vi "test lvjson set.vi"(8 "error in (no error)":errorcluster) -> (0 "error out":errorcluster)   [LabVIEW 2019, in "labview_json_tests.lvlib"]
uses:
  labview_json_tests.lvlib
  lib/Element Set Behavior.ctl
  lib/labview_json.lvlib
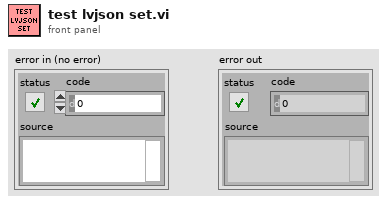
[diagram p1: front panel]
types:
  T1 = typedef "labview_json.lvlib/Element Set Behavior.ctl" = enum8{"Add or Modify", "Modify Only", "Replace"}
  T2 = cluster{"homeTown":string, "formed":i32, "members":cluster{"age":u64}[]}
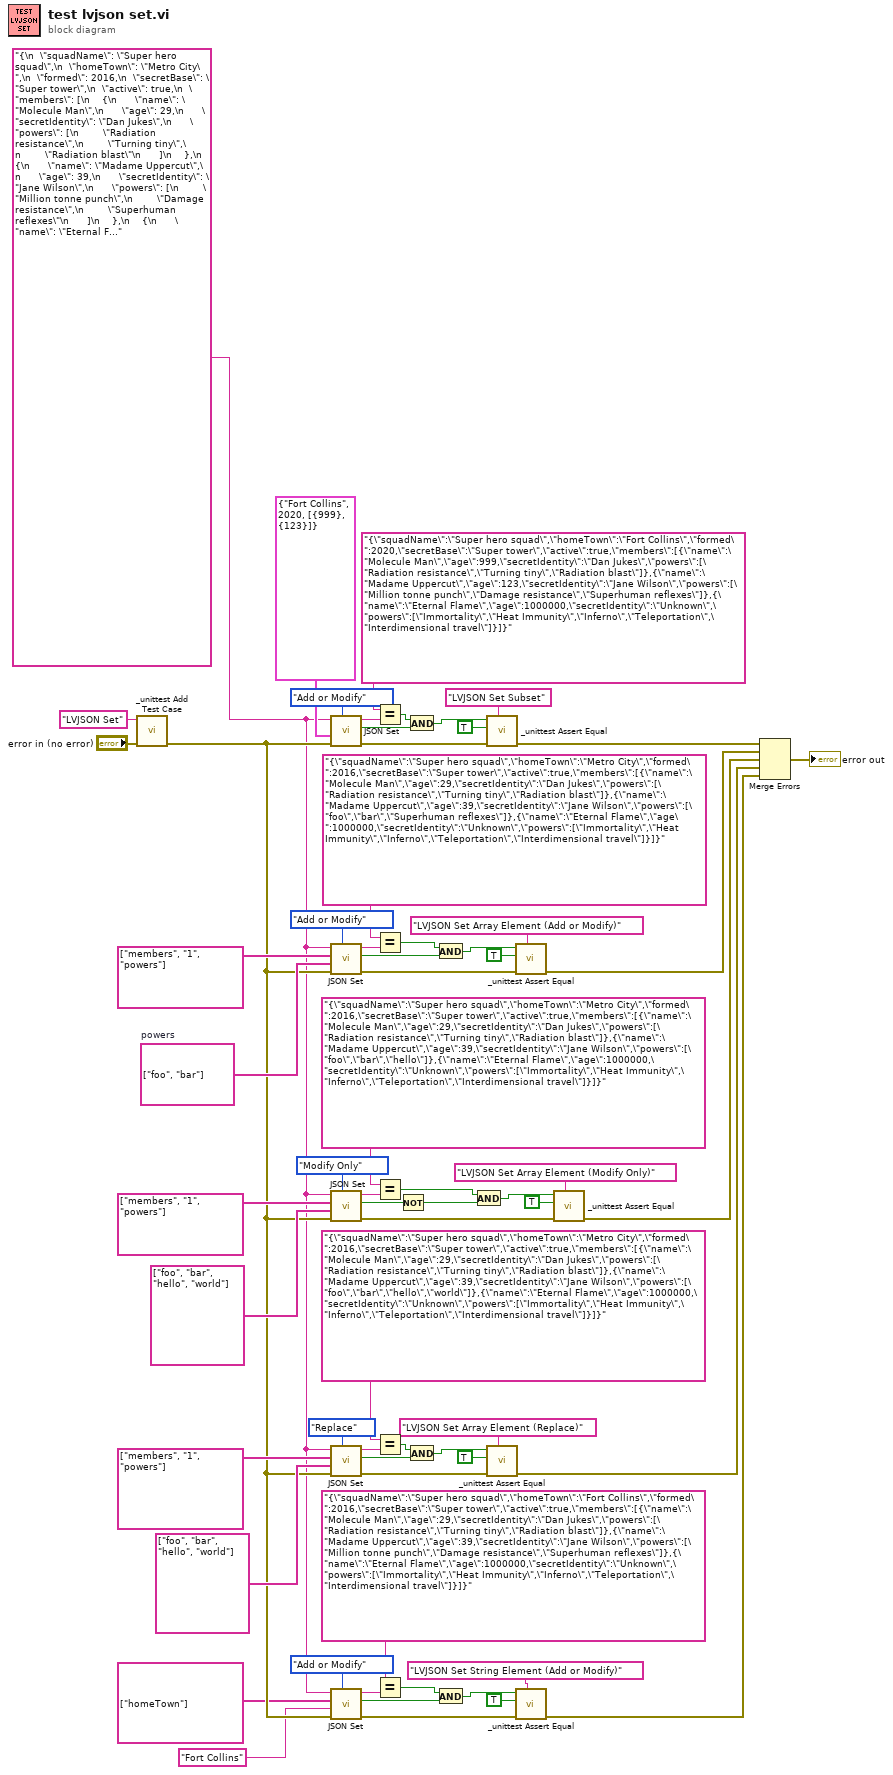
[diagram p0: block diagram]
diagram:
  w15 = string[] ["foo", "bar"]  # powers
  w3 = "{\n  \"squadName\": \"Super hero squad\",\n  \"homeTown\": \"Metro City\",\n  \"formed\": 2016,\n  \"secretBase\": \"Super tower\",\n  \"active\": true,\n  \"members\": [\n    {\n      \"name\": \"Molecule Man\",\n      \"age\": 29,\n      \"secretIdentity\": \"Dan Jukes\",\n      \"powers\": [\n        \"Radiation resistance\",\n        \"Turning tiny\",\n        \"Radiation blast\"\n      ]\n    },\n    {\n      \"name\": \"Madame Uppercut\",\n      \"age\": 39,\n      \"secretIdentity\": \"Jane Wilson\",\n      \"powers\": [\n        \"Million tonne punch\",\n        \"Damage resistance\",\n        \"Superhuman reflexes\"\n      ]\n    },\n    {\n      \"name\": \"Eternal Flame\",\n      \"age\": 1000000,\n      \"secretIdentity\": \"Unknown\",\n      \"powers\": [\n        \"Immortality\",\n        \"Heat Immunity\",\n        \"Inferno\",\n        \"Teleportation\",\n        \"Interdimensional travel\"\n      ]\n    }\n  ]\n}"
  n1 = call "_unittest Add Test Case.vi"("error in (no error)"="error in (no error)", "Test Case"="LVJSON Set") -> ("error out"=w6:errorcluster)  [unwired: 9 in]
  n2 = call "JSON Set.vi"("Behavior (Add or Modify)"=Element_Set_Behavior."Add or Modify", "error in (no error)"=w6, "Value"=T2 {"homeTown"="Fort Collins", "formed"=2020, "members"=[{"age"=999}, {"age"=123}]} ("Root"), "JSON in"=w3) -> ("error out"=w54:errorcluster, "Exists?"=w53:bool, "JSON out"=w56:string)  [unwired: 5 in]
  n3 = call "JSON Set.vi"("Behavior (Add or Modify)"=Element_Set_Behavior."Add or Modify", "error in (no error)"=w6, "Value"=w15, "Root Path ([]=Root)"=string[] ["members", "1", "powers"] ("x"), "JSON in"=w3) -> ("error out"=w51:errorcluster, "Exists?"=w52:bool, "JSON out"=w50:string)  [unwired: 4 in]
  n4 = call "JSON Set.vi"("Behavior (Add or Modify)"=Element_Set_Behavior."Modify Only", "error in (no error)"=w6, "Value"=string[] ["foo", "bar", "hello", "world"], "Root Path ([]=Root)"=string[] ["members", "1", "powers"] ("x"), "JSON in"=w3) -> ("error out"=w32:errorcluster, "Exists?"=w31:bool, "JSON out"=w33:string)  [unwired: 4 in]
  n5 = call "JSON Set.vi"("Behavior (Add or Modify)"=Element_Set_Behavior."Replace", "error in (no error)"=w6, "Value"=string[] ["foo", "bar", "hello", "world"], "Root Path ([]=Root)"=string[] ["members", "1", "powers"] ("x"), "JSON in"=w3) -> ("error out"=w28:errorcluster, "Exists?"=w29:bool, "JSON out"=w27:string)  [unwired: 4 in]
  n6 = call "JSON Set.vi"("Behavior (Add or Modify)"=Element_Set_Behavior."Add or Modify", "error in (no error)"=w6, "Value"="Fort Collins", "Root Path ([]=Root)"=string[] ["homeTown"] ("x"), "JSON in"=w3) -> ("error out"=w8:errorcluster, "Exists?"=w7:bool, "JSON out"=w9:string)  [unwired: 4 in]
  n7 = Equal?(x="{\"squadName\":\"Super hero squad\",\"homeTown\":\"Fort Collins\",\"formed\":2020,\"secretBase\":\"Super tower\",\"active\":true,\"members\":[{\"name\":\"Molecule Man\",\"age\":999,\"secretIdentity\":\"Dan Jukes\",\"powers\":[\"Radiation resistance\",\"Turning tiny\",\"Radiation blast\"]},{\"name\":\"Madame Uppercut\",\"age\":123,\"secretIdentity\":\"Jane Wilson\",\"powers\":[\"Million tonne punch\",\"Damage resistance\",\"Superhuman reflexes\"]},{\"name\":\"Eternal Flame\",\"age\":1000000,\"secretIdentity\":\"Unknown\",\"powers\":[\"Immortality\",\"Heat Immunity\",\"Inferno\",\"Teleportation\",\"Interdimensional travel\"]}]}" ("JSON"), y=w56) -> (x = y?=w59:bool)
  n8 = Equal?(x="{\"squadName\":\"Super hero squad\",\"homeTown\":\"Metro City\",\"formed\":2016,\"secretBase\":\"Super tower\",\"active\":true,\"members\":[{\"name\":\"Molecule Man\",\"age\":29,\"secretIdentity\":\"Dan Jukes\",\"powers\":[\"Radiation resistance\",\"Turning tiny\",\"Radiation blast\"]},{\"name\":\"Madame Uppercut\",\"age\":39,\"secretIdentity\":\"Jane Wilson\",\"powers\":[\"foo\",\"bar\",\"Superhuman reflexes\"]},{\"name\":\"Eternal Flame\",\"age\":1000000,\"secretIdentity\":\"Unknown\",\"powers\":[\"Immortality\",\"Heat Immunity\",\"Inferno\",\"Teleportation\",\"Interdimensional travel\"]}]}" ("JSON"), y=w50) -> (x = y?=w48:bool)
  n9 = Equal?(x="{\"squadName\":\"Super hero squad\",\"homeTown\":\"Metro City\",\"formed\":2016,\"secretBase\":\"Super tower\",\"active\":true,\"members\":[{\"name\":\"Molecule Man\",\"age\":29,\"secretIdentity\":\"Dan Jukes\",\"powers\":[\"Radiation resistance\",\"Turning tiny\",\"Radiation blast\"]},{\"name\":\"Madame Uppercut\",\"age\":39,\"secretIdentity\":\"Jane Wilson\",\"powers\":[\"foo\",\"bar\",\"hello\"]},{\"name\":\"Eternal Flame\",\"age\":1000000,\"secretIdentity\":\"Unknown\",\"powers\":[\"Immortality\",\"Heat Immunity\",\"Inferno\",\"Teleportation\",\"Interdimensional travel\"]}]}" ("JSON"), y=w33) -> (x = y?=w35:bool)
  n10 = Equal?(x="{\"squadName\":\"Super hero squad\",\"homeTown\":\"Metro City\",\"formed\":2016,\"secretBase\":\"Super tower\",\"active\":true,\"members\":[{\"name\":\"Molecule Man\",\"age\":29,\"secretIdentity\":\"Dan Jukes\",\"powers\":[\"Radiation resistance\",\"Turning tiny\",\"Radiation blast\"]},{\"name\":\"Madame Uppercut\",\"age\":39,\"secretIdentity\":\"Jane Wilson\",\"powers\":[\"foo\",\"bar\",\"hello\",\"world\"]},{\"name\":\"Eternal Flame\",\"age\":1000000,\"secretIdentity\":\"Unknown\",\"powers\":[\"Immortality\",\"Heat Immunity\",\"Inferno\",\"Teleportation\",\"Interdimensional travel\"]}]}" ("JSON"), y=w27) -> (x = y?=w25:bool)
  n11 = Equal?(x="{\"squadName\":\"Super hero squad\",\"homeTown\":\"Fort Collins\",\"formed\":2016,\"secretBase\":\"Super tower\",\"active\":true,\"members\":[{\"name\":\"Molecule Man\",\"age\":29,\"secretIdentity\":\"Dan Jukes\",\"powers\":[\"Radiation resistance\",\"Turning tiny\",\"Radiation blast\"]},{\"name\":\"Madame Uppercut\",\"age\":39,\"secretIdentity\":\"Jane Wilson\",\"powers\":[\"Million tonne punch\",\"Damage resistance\",\"Superhuman reflexes\"]},{\"name\":\"Eternal Flame\",\"age\":1000000,\"secretIdentity\":\"Unknown\",\"powers\":[\"Immortality\",\"Heat Immunity\",\"Inferno\",\"Teleportation\",\"Interdimensional travel\"]}]}" ("JSON"), y=w9) -> (x = y?=w11:bool)
  n12 = Not(x=w31) -> (.not. x?=w18:bool)
  n13 = And(x=w59, y=w53) -> (x .and. y?=w57:bool)
  n14 = And(x=w25, y=w29) -> (x .and. y?=w26:bool)
  n15 = And(x=w48, y=w52) -> (x .and. y?=w49:bool)
  n16 = And(x=w11, y=w7) -> (x .and. y?=w10:bool)
  n17 = And(x=w35, y=w18) -> (x .and. y?=w34:bool)
  n18 = call "_unittest Assert Equal.vi"("Message"="LVJSON Set Subset", "error in (no error)"=w54, "Expected Value"=TRUE, "Actual Value"=w57) -> ("error out"=w63:errorcluster)  [unwired: 7 in]
  n19 = call "_unittest Assert Equal.vi"("Message"="LVJSON Set Array Element (Replace)", "error in (no error)"=w28, "Expected Value"=TRUE, "Actual Value"=w26) -> ("error out"=w19:errorcluster)  [unwired: 7 in]
  n20 = call "_unittest Assert Equal.vi"("Message"="LVJSON Set Array Element (Add or Modify)", "error in (no error)"=w51, "Expected Value"=TRUE, "Actual Value"=w49) -> ("error out"=w43:errorcluster)  [unwired: 7 in]
  n21 = call "_unittest Assert Equal.vi"("Message"="LVJSON Set String Element (Add or Modify)", "error in (no error)"=w8, "Expected Value"=TRUE, "Actual Value"=w10) -> ("error out"=w5:errorcluster)  [unwired: 7 in]
  n22 = call "_unittest Assert Equal.vi"("Message"="LVJSON Set Array Element (Modify Only)", "error in (no error)"=w32, "Expected Value"=TRUE, "Actual Value"=w34) -> ("error out"=w30:errorcluster)  [unwired: 7 in]
  n23 = Merge Errors(w63, w43, w30, w19, w5) -> (→"error out":errorcluster)
